vi "CheckForMultiURLs.vi"(8 "error in (no error)":errorcluster, 11 "CS++PVProxy in":refnum<class "CS++PVProxy.lvclass">) -> (0 "error out":errorcluster, 3 "CS++PVProxy out":refnum<class "CS++PVProxy.lvclass">)   [LabVIEW 2016, in "CS++PVProxy.lvlib" / "CS++PVProxy.lvclass"]
doc: "This VI checks if mor ethan one URL is present in the \"PV URL\" attribute and if yes, they are seperated in different array entries."
uses:
  CS++PVProxy.lvclass
  CS++PVProxy.lvclass/CS++PVProxy.ctl
  CS++PVMonitor Messages/CS++PVUpdate Msg/CS++PVUpdate Msg.lvclass/CS++PVUpdate Msg.ctl
  Classes/CS++ProcessVariables/ProcessVariable/PV.lvclass/PV.ctl
  <vilib>/Utility/error.llb/Error Cluster From Error Code.vi
  CS++PVMonitor Messages/CS++PVUpdate Msg/CS++PVUpdate Msg.lvclass
  Classes/CS++ProcessVariables/PVConnection/PVConnection.lvclass
  Classes/CS++ProcessVariables/ProcessVariable/PV.lvclass
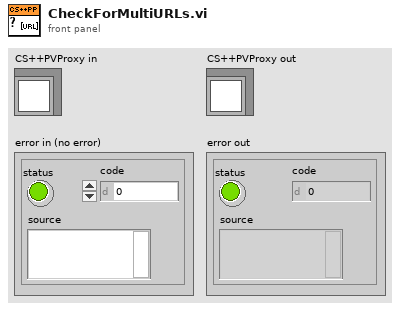
[diagram p1: front panel]
types:
  T1 = cluster{"Name":string, "Polling-String":string, "CS++PVUpdate Msg":refnum<class "CS++PVUpdate Msg.lvclass">, "PVConnection":refnum<class "PVConnection.lvclass">}[]
  T2 = cluster{"Name":string, "Polling-String":string, "CS++PVUpdate Msg":refnum<class "CS++PVUpdate Msg.lvclass">, "PVConnection":refnum<class "PVConnection.lvclass">}
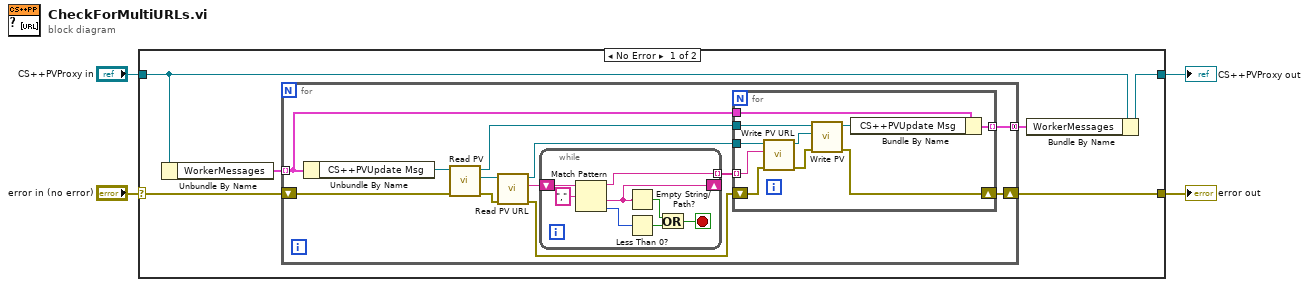
[diagram p0: block diagram]
diagram:
  n1 = case shown="No Error" "error in (no error)" {
    selector: "error in (no error)" -> [w6 w42]
    tunnel: [w5 w42] -> w3
    tunnel: [w8 w41] -> w1
    tunnel: "CS++PVProxy in" -> [w10 w41]
    frame No Error {
      n2 = Unbundle By Name(w10) -> ("WorkerMessages"=w9:T1)
      n3 = for {
        tunnel: w9 -> [w15] mode=indexing
        tunnel: [w14] -> w7 mode=concatenating
        shift-right: [w11] -> w5
        shift-left: w6 -> [w13]
        n4 = Unbundle By Name(w15) -> ("CS++PVUpdate Msg"=w22:refnum<class "CS++PVUpdate Msg.lvclass">)
        n5 = call "Read PV.vi"("error in (no error)"=w13, "CS++PVUpdate Msg in"=w22) -> ("error out"=w19:errorcluster, "PV"=w21:refnum<class "PV.lvclass">, "CS++PVUpdate Msg out"=w16:refnum<class "CS++PVUpdate Msg.lvclass">)  [unwired: 7 in]
        n6 = call "Read PV URL.vi"("error in (no error)"=w19, "PV in"=w21) -> ("error out"=w12:errorcluster, "PV URL"=w20:string, "PV out"=w18:refnum<class "PV.lvclass">)  [unwired: 7 in]
        n7 = while {
          shift-right: [w35] -> _
          shift-left: w20 -> [w40]
          tunnel: [w33] -> w17 mode=indexing
          stop <- w37 stop-if-true
          n8 = Match Pattern(string=w40, regular expression=",") -> (before substring=w33:string, after substring=w35:string, offset past match=w38:i32)  [unwired: 1 in, 1 out]
          n9 = Empty String/Path?(string/path=w35) -> (empty?=w34:bool)
          n10 = Less Than 0?(x=w38) -> (x < 0?=w36:bool)
          n11 = Or(x=w34, y=w36) -> (x .or. y?=w37:bool)
        }
        n12 = for {
          tunnel: w18 -> [w32]
          tunnel: w17 -> [w31] mode=indexing
          tunnel: w16 -> [w30]
          tunnel: w15 -> [w27]
          tunnel: [w25] -> w14 mode=indexing
          shift-right: [w23] -> w11
          shift-left: w12 -> [w24]
          n13 = call "Write PV URL.vi"("error in (no error)"=w24, "PV URL"=w31, "PV in"=w32) -> ("error out"=w28:errorcluster, "PV out"=w29:refnum<class "PV.lvclass">)  [unwired: 7 in]
          n14 = call "Write PV.vi"("error in (no error)"=w28, "PV"=w29, "CS++PVUpdate Msg in"=w30) -> ("error out"=w23:errorcluster, "CS++PVUpdate Msg out"=w26:refnum<class "CS++PVUpdate Msg.lvclass">)  [unwired: 7 in]
          n15 = Bundle By Name(cluster=w27, "CS++PVUpdate Msg"=w26) -> (w25:T2)
        }
      }
      n16 = Bundle By Name(cluster=w10, "WorkerMessages"=w7) -> (w8:refnum<class "CS++PVProxy.lvclass">)
    }
    frame Error {
    }
  }
  "error out" <- w3
  "CS++PVProxy out" <- w1
